vi "Update Map.vi"(8 "error in (no error)":errorcluster, 10 "Team Map":i32[][](array[numeric]), 11 "Team Field Panel in":refnum<class "Team Field Panel.lvclass">) -> (0 "error out":errorcluster, 3 "Team Field Panel out":refnum<class "Team Field Panel.lvclass">)   [LabVIEW 2020, in "SB App.lvlib" / "Team Field Panel.lvclass"]
uses:
  Team Field Panel.lvclass
  Team Map Update Data.ctl
  Team Field Panel.lvclass/Team Field Panel.ctl
  SB App.lvlib
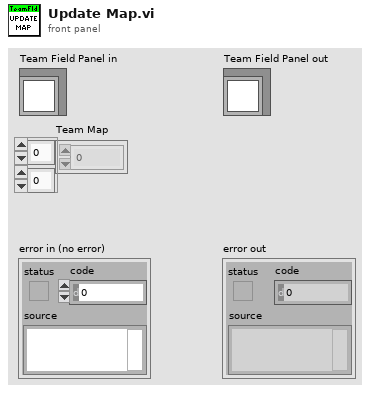
[diagram p1: front panel]
types:
  T1 = typedef "SB App.lvlib/Team Map Update Data.ctl" = cluster{"Team Map":i32[][]}
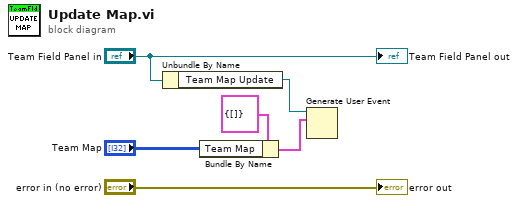
[diagram p0: block diagram]
diagram:
  n1 = Unbundle By Name("Team Field Panel in") -> ("Team Map Update"=w4:refnum<user-event>)
  n2 = Bundle By Name(cluster=T1 {"Team Map"=[]} ("event data"), "Team Map"="Team Map") -> (w2:T1)
  n3 = Generate User Event(user event=w4, event data cluster=w2) -> ()  [unwired: 2 in, 2 out]
  "error out" <- "error in (no error)"
  "Team Field Panel out" <- "Team Field Panel in"
